vi "commonMotionMove.vi"(6 "timeout":dbl=-1.0, 7 "line move mode":i32(ring)=10551337 items=["Relative"=10551344, "Absolute"=10551337, "Relative To Capture"=10551345, "Velocity"=10551346, "Polyline"=11600101], 8 "error in":errorcluster, 9 "velocity":dbl=1000.0, 10 "position":dbl=1000.0, 11 "resource":refnum<k21>) -> (0 "error out":errorcluster, 2 "timed out?":bool, 3 "resource out":refnum<k21>)   [LabVIEW 2018]
uses:
  <vilib>/Motion/PropertyNodes/nimc.createStraightLineMoveInstance.axis.vi
  <vilib>/Motion/PropertyNodes/nimc.waitUntilDone.straightLineMove.vi
  <resource>/objmgr/nimotion.rc
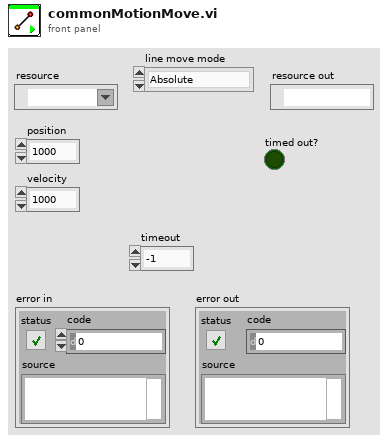
[diagram p1: front panel]
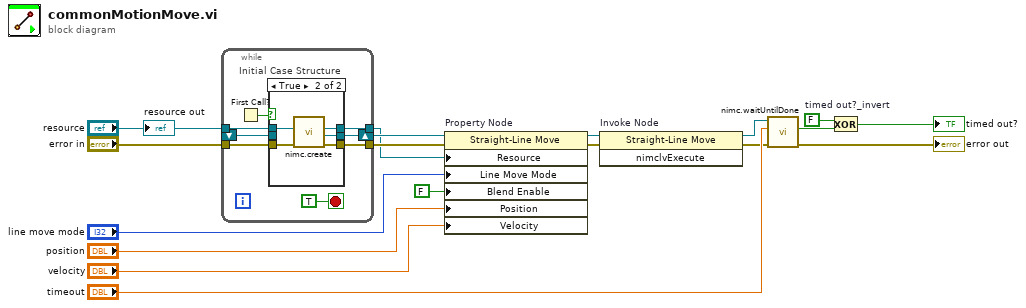
[diagram p0: block diagram]
diagram:
  w15 = FALSE  # timed out?_invert
  n1 = while {
    tunnel: "resource" -> [w26]
    tunnel: "error in" -> [w24]
    tunnel: [w23] -> w11
    shift-right: [w25] -> w10
    shift-left: _ -> [w21]
    tunnel: [w19] -> w1
    stop <- TRUE stop-if-true
    n2 = First Call?() -> (First Call?: T/F=w20:bool)
    n3 = case "Initial Case Structure" shown="True" w20 {
      tunnel: w26 -> [w27 w32]
      tunnel: [w28 w31] -> w25
      tunnel: w24 -> [w29 w33]
      tunnel: [w29 w34] -> w23
      tunnel: w21 -> [w28 _]
      tunnel: [w27 w30] -> w19
      frame False {
      }
      frame True {
        n4 = call-poly <vilib>:"nimc.create.vi"("error in"=w33, "axis"=w32) -> ("error out"=w34:errorcluster, "axis out"=w30:refnum<k21>, "line"=w31:refnum<k20>)  [unwired: 7 in]
      }
    }
  }
  n5 = property on="Property Node" class="Straight-Line Move"(reference=w10, error in=w11, "Resource"=w1, "Line Move Mode"="line move mode", "Blend Enable"=FALSE ("blend enable"), "Position"="position", "Velocity"="velocity") -> (reference out=w9:refnum<k20>, error out=w8:errorcluster)
  n6 = invoke on="Invoke Node" class="Straight-Line Move" method="nimclvExecute"(reference=w9, error in=w8) -> (reference out=w13:refnum<k20>, error out=w12:errorcluster)  [unwired: 1 in, 1 out]
  n7 = call-poly <vilib>:"nimc.waitUntilDone.vi"("error in"=w12, "timeout"="timeout", "motion handle"=w13) -> ("error out"=→"error out":errorcluster, "timed out?"=w16:bool)  [unwired: 6 in, 1 out]
  n8 = Exclusive Or(1:w16, 2:w15) -> (0:→"timed out?":bool)
  "resource out" <- "resource"
